vi "Array to Ring.vi"(11 "Array In":string[](array[string])) -> (3 "Name Ring Out":u16(ring) items=["Chris", "Derek", "Jeremy", "Joshua", "Katelyn", "Loah", "Oana", "Pete"])   [LabVIEW 2011]
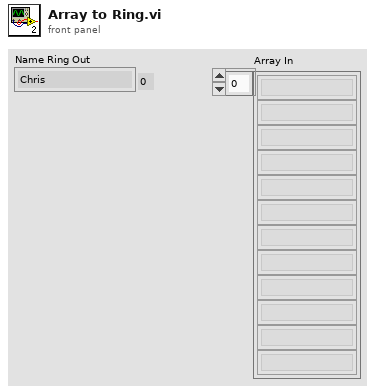
[diagram p1: front panel]
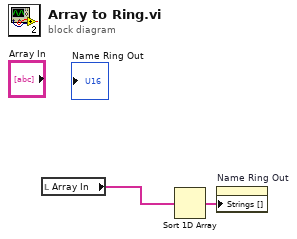
[diagram p0: block diagram]
diagram:
  n1 = local read "Array In"() -> (w1:string[])
  n2 = Sort 1D Array(array=w1) -> (sorted array=w2:string[])
  n3 = property on="Name Ring Out" class="Ring (strict)"("Strings []"=w2) -> ()  [unwired: 2 in, 2 out]
